vi "ws Application Folder.vi"(3 "Relative Path (\"\" - Folder)":string) -> (1 "Application Folder":path)   [LabVIEW 2011]
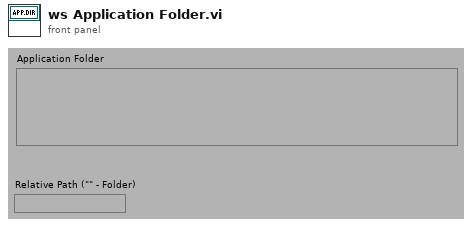
[diagram p1: front panel]
types:
  T1 = enum32{"invalid app kind", "Development System", "Run Time System", "Student Edition", "Embedded LabVIEW", "Evaluation", "Custom"}
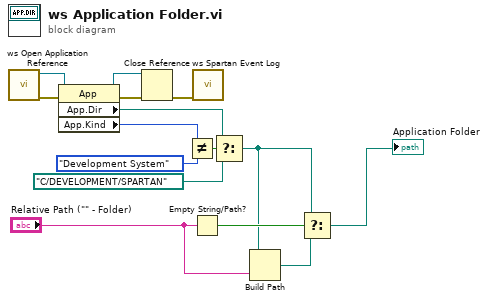
[diagram p0: block diagram]
diagram:
  n1 = call "ws Open Application Reference.vi"() -> ("error out"=w3:errorcluster, "application reference"=w2:refnum<vi>)  [unwired: 10 in]
  n2 = property class="App"(reference=w2, error in=w3) -> (reference out=w9:refnum<vi>, error out=w10:errorcluster, "App.Dir"=w7:path, "App.Kind"=w5:T1)
  n3 = Close Reference(reference=w9, error in (no error)=w10) -> (error out=w1:errorcluster)
  n4 = Not Equal?(x=w5, y=T1."Development System") -> (x != y?=w8:bool)
  n5 = Empty String/Path?(string/path="Relative Path (\"\" - Folder)") -> (empty?=w13:bool)
  n6 = call "ws Spartan Event Log.vi"("error in (no error)"=w1) -> ()  [unwired: 7 in, 1 out]
  n7 = Select(t=w7, s=w8, f=path "C:/DEVELOPMENT/SPARTAN" ("start path")) -> (s? t:f=w6:path)
  n8 = Build Path(base path=w6, name or relative path="Relative Path (\"\" - Folder)") -> (appended path=w12:path)
  n9 = Select(t=w6, s=w13, f=w12) -> (s? t:f=→"Application Folder":path)
